vi "XML Reader Start Root.vi"(8 "error in":errorcluster, 10 "Root Name":string="Calibration", 11 "XML Reader In":T1) -> (0 "error out":errorcluster, 3 "XML Reader Out":T1)   [LabVIEW 2018, in "Pathloss XML Reader.lvlib"]
uses:
  Pathloss XML Reader.lvlib
  Controls/XML Reader Data Ref.ctl
  Controls/XML Reader Data.ctl
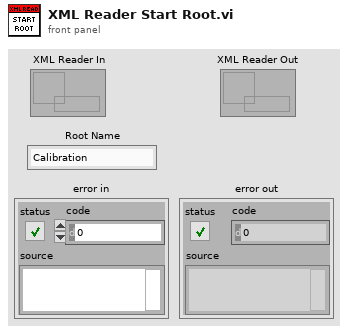
[diagram p1: front panel]
types:
  T1 = typedef "Pathloss XML Reader.lvlib/XML Reader Data Ref.ctl" = refnum<data-value>
  T2 = typedef "Pathloss XML Reader.lvlib/XML Reader Data.ctl" = cluster{"Remaining XML":string, "Section Name Stack":string[], "Section Stack":string[]}
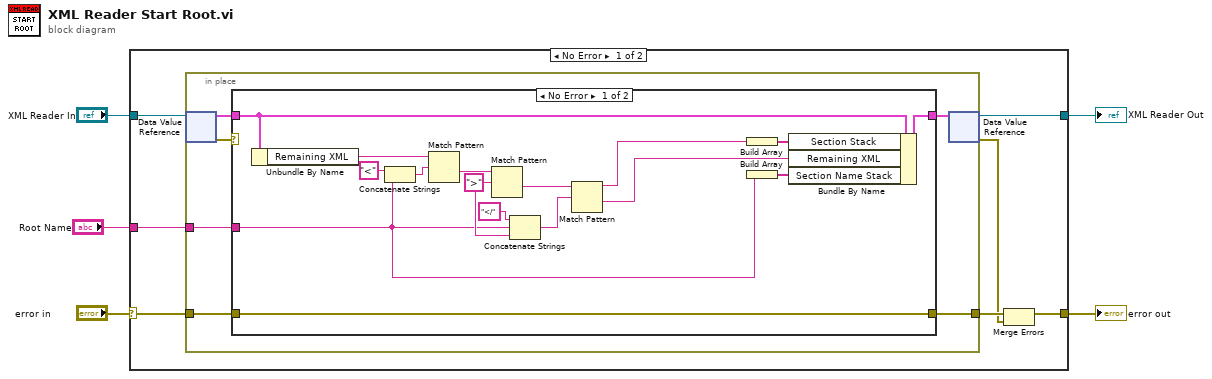
[diagram p0: block diagram]
diagram:
  n1 = case shown="No Error" "error in" {
    selector: "error in" -> [w10 w37]
    tunnel: [w7 w37] -> w5
    tunnel: [w11 w38] -> w4
    tunnel: "XML Reader In" -> [w12 w38]
    tunnel: "Root Name" -> [w8 _]
    frame No Error {
      n2 = in-place {
        in-place-border: w10 -> [w15]
        in-place-border: [w14] -> w9
        in-place-border: w8 -> [w13]
        n3 = in-place-dvr #1(w12) -> (w17:T2, w18:errorcluster)
        n4 = case shown="No Error" w18 {
          selector: w18 -> [_ w35]
          tunnel: w17 -> [w34 w36]
          tunnel: [w33 w36] -> w16
          tunnel: w15 -> [w29 _]
          tunnel: [w29 w35] -> w14
          tunnel: w13 -> [w24 _]
          frame No Error {
            w28 = ">" ("regular expression")
            n5 = Unbundle By Name(w34) -> ("Remaining XML"=w26:string)
            n6 = Concatenate Strings("<" ("string"), w24) -> (w31:string)
            n7 = Match Pattern(string=w26, regular expression=w31) -> (after substring=w30:string)  [unwired: 1 in, 3 out]
            n8 = Match Pattern(string=w30, regular expression=w28) -> (after substring=w22:string)  [unwired: 1 in, 3 out]
            n9 = Concatenate Strings("</" ("string"), w24, w28) -> (w21:string)
            n10 = Match Pattern(string=w22, regular expression=w21) -> (before substring=w20:string, after substring=w19:string)  [unwired: 1 in, 2 out]
            n11 = Build Array(w20) -> (w23:string[])
            n12 = Build Array(w24) -> (w25:string[])
            n13 = Bundle By Name(cluster=w34, "Section Stack"=w23, "Remaining XML"=w19, "Section Name Stack"=w25) -> (w33:T2)
          }
          frame Error {
          }
        }
        n14 = in-place-dvr #1(w16) -> (w11:T1, w6:errorcluster)
      }
      n15 = Merge Errors(w9, w6) -> (w7:errorcluster)
    }
    frame Error {
    }
  }
  "error out" <- w5
  "XML Reader Out" <- w4
